vi "Hist_Xo_and_Delta_X.vi"(2 "Histogram index":i32) -> (5 "Xo":dbl format="%.2f", 6 "Delta X":dbl format="%.2f")   [LabVIEW 2010]
uses:
  Globals/Meas_global.vi
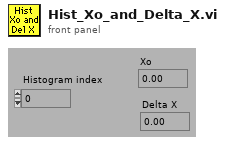
[diagram p1: front panel]
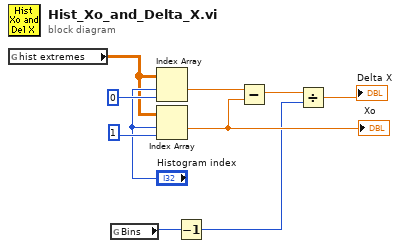
[diagram p0: block diagram]
diagram:
  n1 = global read "Meas_global.vi" "hist extremes"() -> (w7:dbl[][])
  n2 = global read "Meas_global.vi" "Bins"() -> (w4:i32)
  n3 = Index Array(array=w7, index (row)="Histogram index", index (col)=0) -> (element=w6:dbl)
  n4 = Index Array(array=w7, index (row)="Histogram index", index (col)=1) -> (element=w5:dbl)
  "Xo" <- w5
  n5 = Decrement(x=w4) -> (x-1=w2:i32)
  n6 = Subtract(x=w6, y=w5) -> (x-y=w3:dbl)
  n7 = Divide(x=w3, y=w2) -> (x/y=→"Delta X":dbl)
